vi "PositionNet.vi"() -> ()   [LabVIEW 2016]
uses:
  <vilib>/Analysis/baseanly.llb/A x Vector.vi
  <vilib>/Analysis/NI_AALBase.lvlib
panel:
  out "Numeric 3":dbl
  out "Array 3":dbl[](array[numeric])
  in  "Array":dbl[](array[numeric])
  out "Numeric":dbl
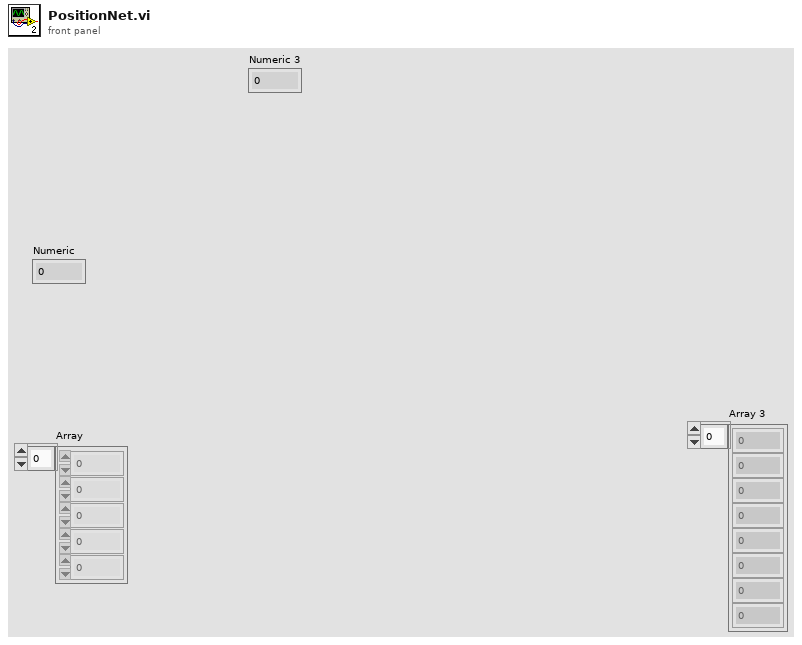
[diagram p1: front panel]
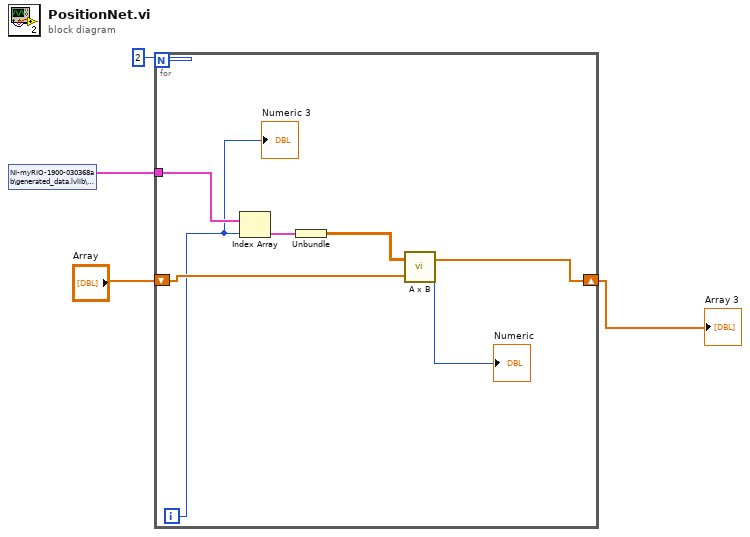
[diagram p0: block diagram]
diagram:
  n1 = shared-variable "NI-myRIO-1900-030368ab\\generated_data.lvlib\\Weights"() -> (w4:cluster{"all rows":dbl[][]}[])  [unwired: 1 in, 1 out]
  n2 = for {
    N: 2 -> [_]
    tunnel: w4 -> [w11]
    shift-right: [w8] -> w2
    shift-left: "Array" -> [w7]
    i -> [w6]
    n3 = Index Array(array=w11, index=w6) -> (element=w10:cluster{"all rows":dbl[][]})
    n4 = Unbundle(w10) -> ("all rows"=w5:dbl[][])
    n5 = call-poly <vilib>:"A x B.vi"("Vector"=w7, "A"=w5) -> ("error"=→"Numeric":i32, "A x Vector"=w8:dbl[])
    "Numeric 3" <- w6
  }
  "Array 3" <- w2
